vi "ULx Write (Digital 1D Wfm NChan 1Samp).vi"(0 "task in":refnum<k24>, 1 "auto start":bool, 7 "data":digitalwaveform[](array[waveform]), 9 "timeout":dbl=10.0 format="%_4g", 11 "error in":errorcluster) -> (4 "task out":refnum<k24>, 10 "number of samples written per channel":u32, 15 "error out":errorcluster)   [LabVIEW 2020]
doc: "Writes a digital waveform that contains a single sample to each channel in a task that contains one or more digital output channels."
uses:
  C:/Users/William/Documents/LV 2020 builds/LeaktestDAQ/Source-v33/ULx_LV.dll
  ULx_LV.dll
panel:
  # "channel"
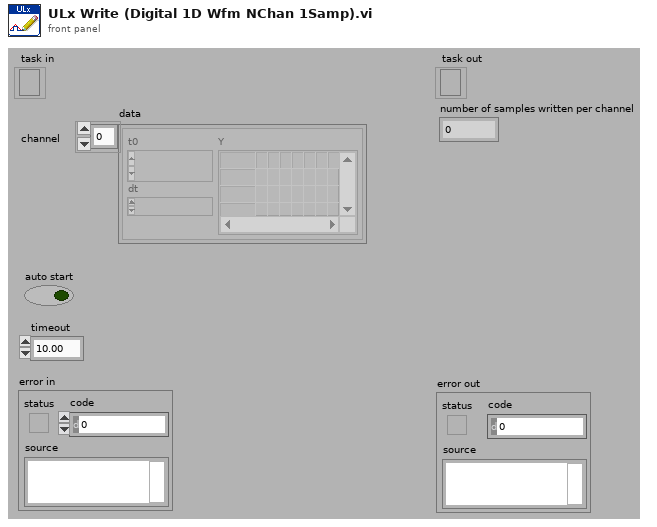
[diagram p1: front panel]
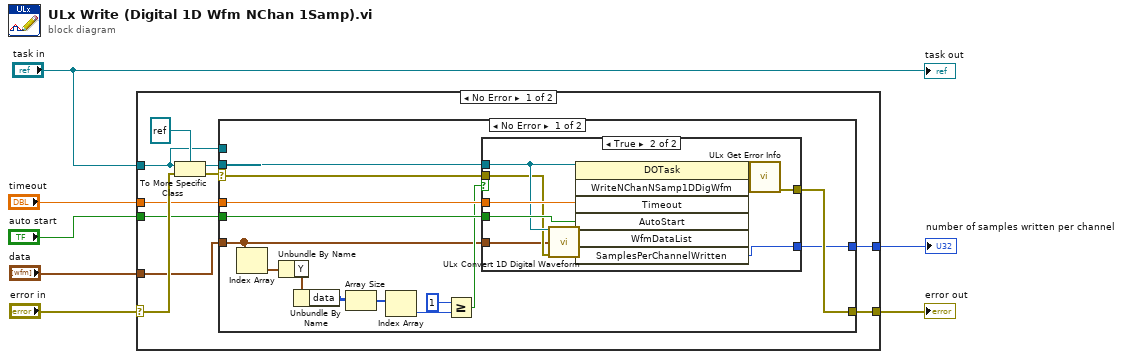
[diagram p0: block diagram]
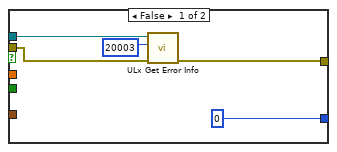
[diagram p2: hidden frame]
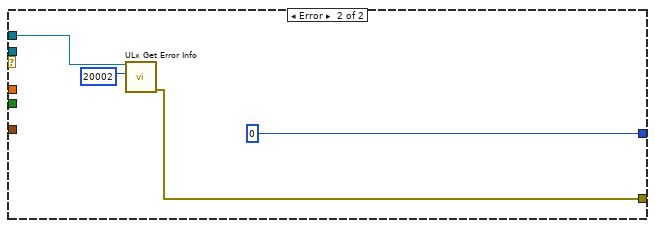
[diagram p3: hidden frame]
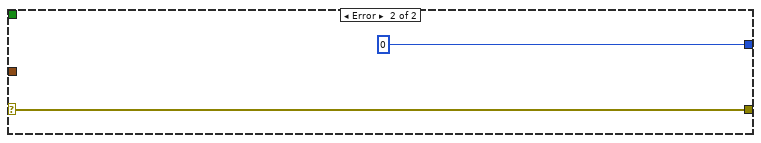
[diagram p4: hidden frame]
diagram:
  n1 = case shown="No Error" "error in" {
    selector: "error in" -> [w17 w53]
    tunnel: "task in" -> [w11 _]
    tunnel: "timeout" -> [w13 _]
    tunnel: [w12 w53] -> w5
    tunnel: "auto start" -> [w10 _]
    tunnel: [w9 0 ("SamplesPerChannelWritten")] -> w2
    tunnel: "data" -> [w8 _]
    frame No Error {
      n2 = To More Specific Class(target class=refnum<k24> refnum, reference=w11, error in=w17) -> (specific class reference=w14:refnum<k24>, error out=w15:errorcluster)
      n3 = case shown="No Error" w15 {
        selector: w15 -> [w26 _]
        tunnel: w14 -> [w27 _]
        tunnel: w13 -> [w29 _]
        tunnel: [w31 w50] -> w12
        tunnel: w11 -> [_ w49]
        tunnel: w10 -> [w28 _]
        tunnel: [w30 0 ("SamplesPerChannelWritten")] -> w9
        tunnel: w8 -> [w19 _]
        frame No Error {
          n4 = Index Array(array=w19) -> (element=w18:digitalwaveform)  [unwired: 1 in]
          n5 = Unbundle By Name(w18) -> ("Y"=w22:digitaldata)
          n6 = Unbundle By Name(w22) -> ("data"=w25:u8[][])
          n7 = Array Size(array=w25) -> (size(s)=w24:i32[])
          n8 = Index Array(array=w24) -> (element=w21:i32)  [unwired: 1 in]
          n9 = Greater Or Equal?(x=1 ("y"), y=w21) -> (x >= y?=w23:bool)
          n10 = case shown="True" w23 {
            tunnel: [w33 w45] -> w31
            tunnel: [u32 0 ("SamplesPerChannelWritten") w43] -> w30
            tunnel: w29 -> [_ w42]
            tunnel: w28 -> [_ w41]
            tunnel: w27 -> [w35 w40]
            tunnel: w26 -> [w34 w39]
            tunnel: w19 -> [_ w37]
            frame False {
              n11 = call "ULx Get Error Info.vi"("error in"=w34, "ErrorCode"=20003, "task in"=w35) -> ("error out"=w33:errorcluster)  [unwired: 8 in]
            }
            frame True {
              n12 = call "ULx Convert 1D Digital Waveform.vi"("task in"=w40, "data"=w37, "error in"=w39) -> ("data List"=w38:refnum<k24>)  [unwired: 11 in, 1 out]
              n13 = invoke class="DOTask" method="WriteNChanNSamp1DDigWfm"(reference=w40, "Timeout"=w42, "AutoStart"=w41, "WfmDataList"=w38) -> (reference out=w46:refnum<k24>, error out=w47:errorcluster, "WriteNChanNSamp1DDigWfm"=w44:i32, "SamplesPerChannelWritten"=w43:u32)  [unwired: 3 in, 3 out]
              n14 = call "ULx Get Error Info.vi"("error in"=w47, "ErrorCode"=w44, "task in"=w46) -> ("error out"=w45:errorcluster)  [unwired: 8 in]
            }
          }
        }
        frame Error {
          n15 = call "ULx Get Error Info.vi"("ErrorCode"=20002, "task in"=w49) -> ("error out"=w50:errorcluster)  [unwired: 9 in]
        }
      }
    }
    frame Error {
    }
  }
  "error out" <- w5
  "number of samples written per channel" <- w2
  "task out" <- "task in"
